vi "TomsToolsDocumentationTool_Provider_InitItems.vi"(11 "objects":T1[](array[typedef])) -> ()   [LabVIEW 2015]
uses:
  <resource>/Framework/Providers/API/ItemRef.ctl
panel:
  out "error out":errorcluster
  in  "error in":errorcluster
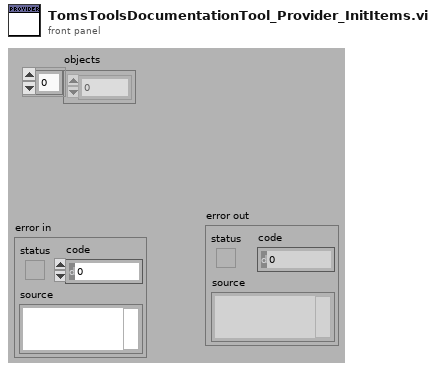
[diagram p1: front panel]
types:
  T1 = typedef "ItemRef.ctl" = u64
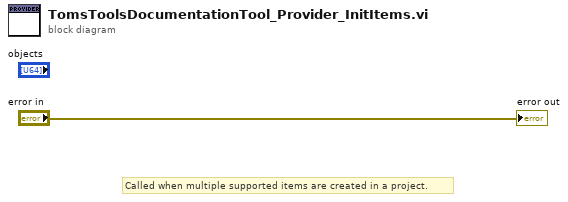
[diagram p0: block diagram]
diagram:
  # "Called when multiple supported items are created in a project."
  "error out" <- "error in"
